vi "dlc 2 length.vi"(1 "dlc":i32) -> (0 "length":i32)   [LabVIEW 2024, in "atsj peakcan basic.lvlib"]
uses:
  atsj peakcan basic.lvlib
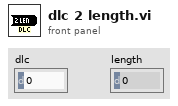
[diagram p1: front panel]
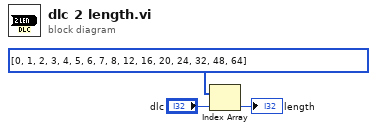
[diagram p0: block diagram]
diagram:
  n1 = Index Array(array=i32[] [0, 1, 2, 3, 4, 5, 6, 7, 8, 12, 16, 20, 24, 32, 48, 64], index="dlc") -> (element=→"length":i32)
